vi "Update Timer Data.vi"(5 "Timer Data for timer in":T1={"Protocol Timer State"=enum."Start", "Remaining session time"=0.0, "Curent interval duration"=0.0, "Time of last iteration"=0.0, "Time elapsed in current iteration"=0.0, "Current interval indicator"=[], "Current interval index"=0, "Time to next interval"=0.0, "Protocol"=[]}) -> (1 "Interval up?":bool, 2 "Timer Data for timer out":T1={"Protocol Timer State"=enum."Start", "Remaining session time"=0.0, "Curent interval duration"=0.0, "Time of last iteration"=0.0, "Time elapsed in current iteration"=0.0, "Current interval indicator"=[], "Current interval index"=0, "Time to next interval"=0.0, "Protocol"=[]})   [LabVIEW 2019]
uses:
  Controls/Timer Data for timer.ctl
  Version 2/States/Protocol Timer States.ctl
  Controls/Protocol Interval.ctl
  Controls/Stim Interval Mode.ctl
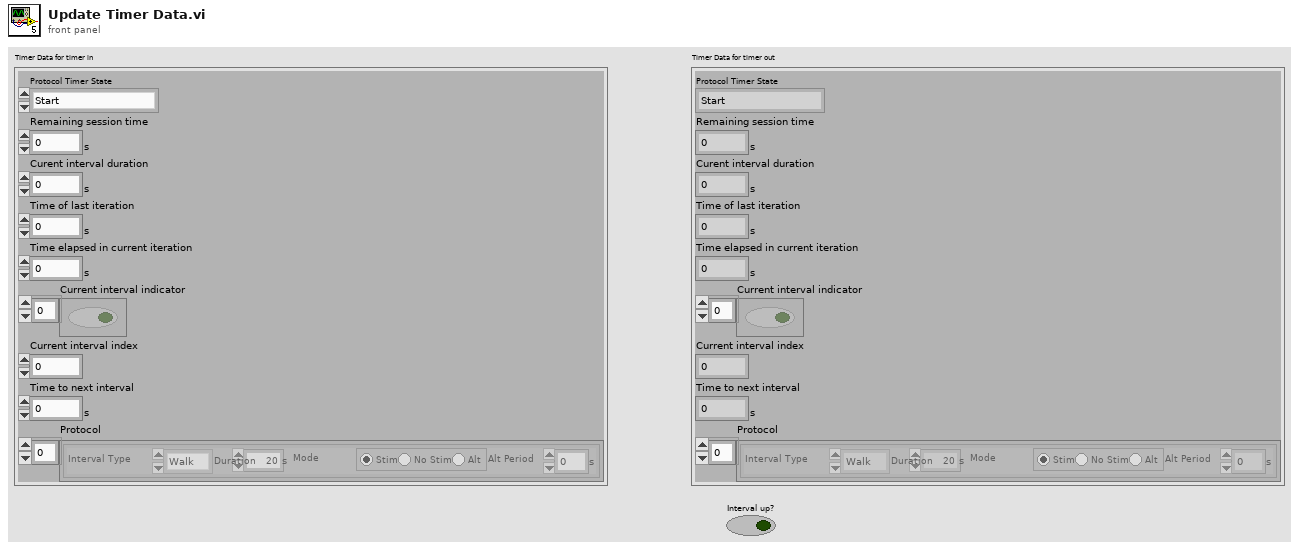
[diagram p1: front panel]
types:
  T1 = typedef "Timer Data for timer.ctl" = cluster{"Protocol Timer State":T2, "Remaining session time":dbl[unit], "Curent interval duration":dbl[unit], "Time of last iteration":dbl[unit], "Time elapsed in current iteration":dbl[unit], "Current interval indicator":bool[], "Current interval index":u32, "Time to next interval":dbl[unit], "Protocol":T3[]}
  T2 = typedef "Protocol Timer States.ctl" = enum16{"Initialize", "Start", "Advance", "Stop", "Pause", "Resume", "Reset"}
  T3 = typedef "Protocol Interval.ctl" = cluster{"Interval Type":enum16{"Walk", "Rest"}, "Duration":dbl[unit], " Mode":T4, "Alt Period":dbl[unit]}
  T4 = typedef "Stim Interval Mode.ctl" = enum32{"Stim", "No Stim", "Alternating"}
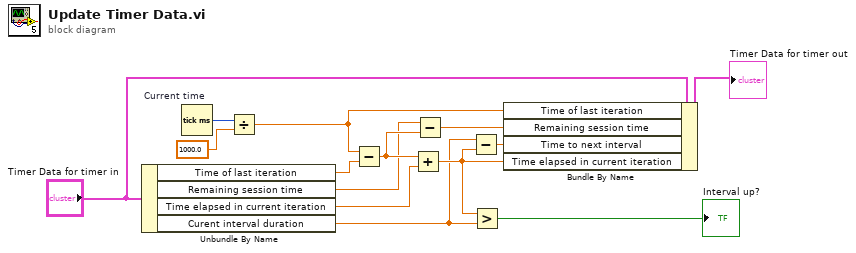
[diagram p0: block diagram]
diagram:
  n1 = Unbundle By Name("Timer Data for timer in") -> ("Time of last iteration"=w6:dbl[unit], "Remaining session time"=w5:dbl[unit], "Time elapsed in current iteration"=w11:dbl[unit], "Curent interval duration"=w13:dbl[unit])
  n2 = Tick Count (ms) "Current time"() -> (millisecond timer value=w3:u32)
  n3 = Divide(x=w3, y=dbl[unit] 1000.0) -> (x/y=w1:dbl[unit])
  n4 = Subtract(x=w1, y=w6) -> (x-y=w12:dbl[unit])
  n5 = Add(x=w12, y=w11) -> (x+y=w14:dbl[unit])
  n6 = Subtract(x=w5, y=w12) -> (x-y=w8:dbl[unit])
  n7 = Subtract(x=w13, y=w14) -> (x-y=w9:dbl[unit])
  n8 = Greater?(x=w14, y=w13) -> (0:→"Interval up?":bool)
  n9 = Bundle By Name(cluster="Timer Data for timer in", "Time of last iteration"=w1, "Remaining session time"=w8, "Time to next interval"=w9, "Time elapsed in current iteration"=w14) -> (→"Timer Data for timer out":T1)
